vi "TrafficLight.vi"() -> ()   [LabVIEW 2018]
panel:
  in  "Car Waiting NS":bool
  in  "Car Waiting EW":bool
  in  "Light Time":sgl(slide)=1.0 min=1 max=30 step=1 scale=1.0..30.0
  in  "Flashing Red":bool
  in  "Emergency":bool
  out "NS2 G":bool
  out "NS2 Y":bool
  out "NS2 R":bool
  out "EW2 G":bool
  out "EW2 Y":bool
  out "EW2 R":bool
  out "NS1 G":bool
  out "NS1 Y":bool
  out "NS1 R":bool
  out "EW1 G":bool
  out "EW1 Y":bool
  out "EW1 R":bool
  in  "stop":bool
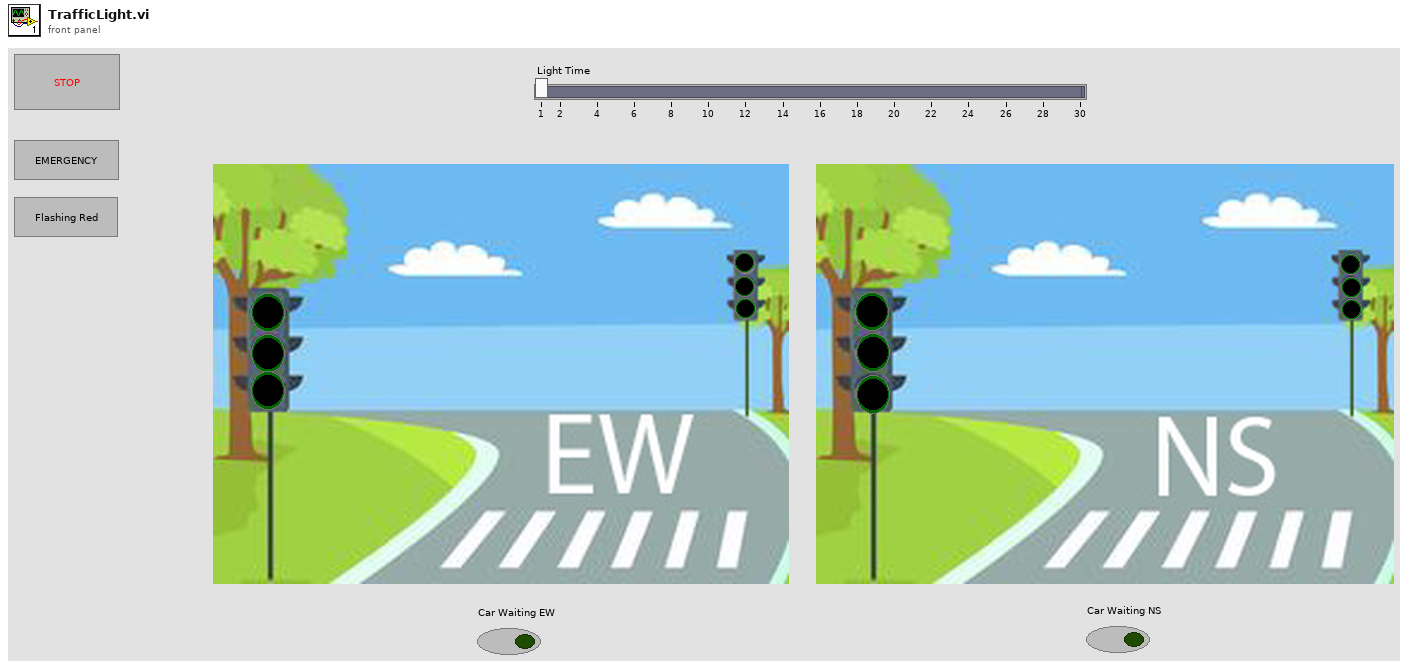
[diagram p1: front panel]
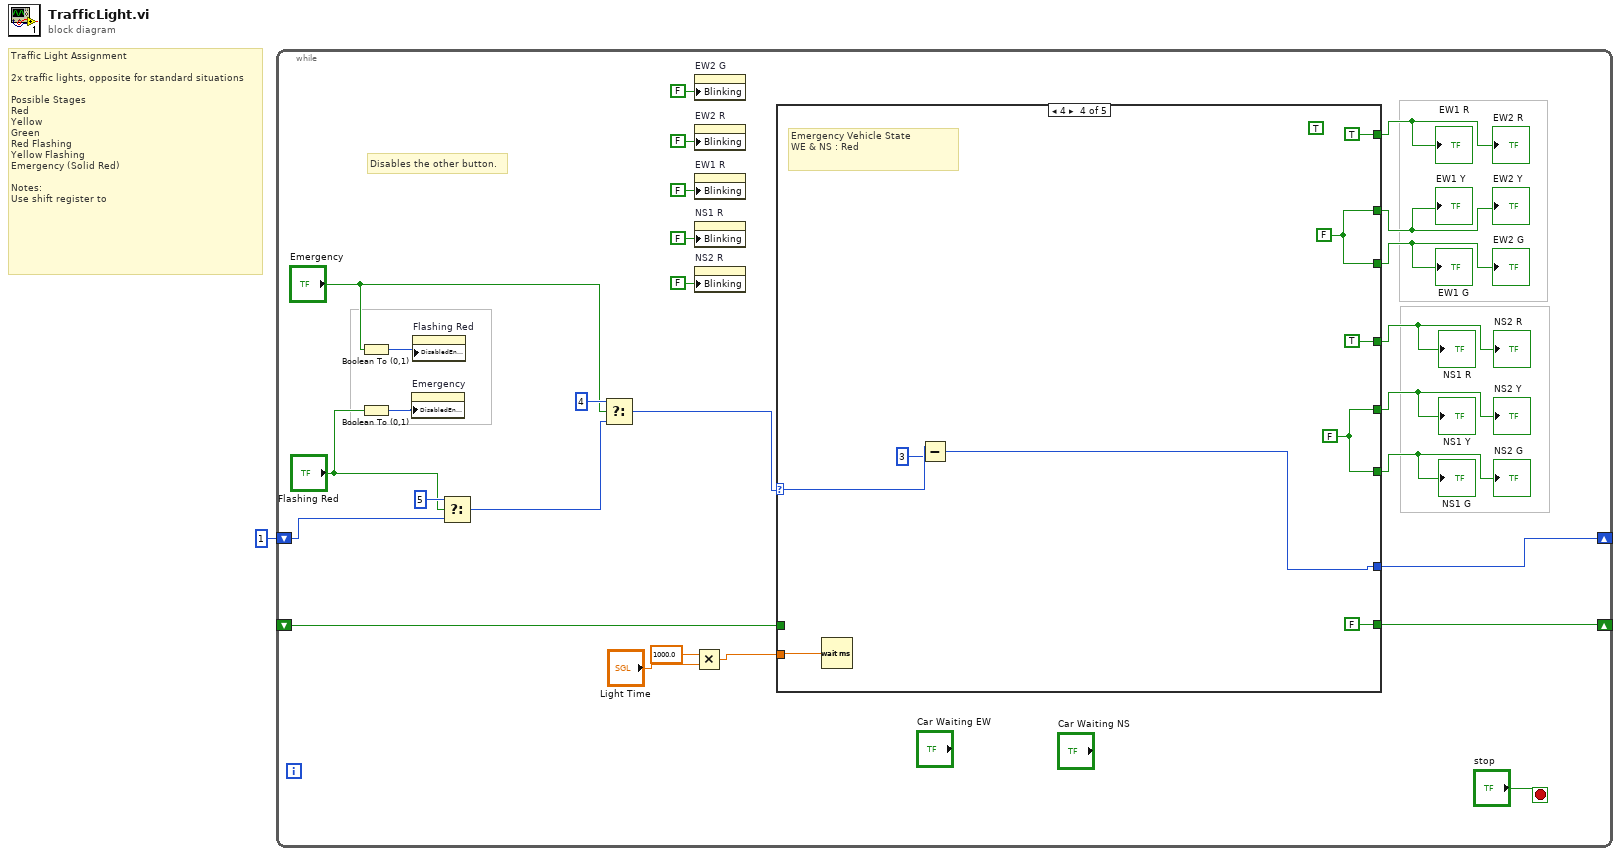
[diagram p0: block diagram]
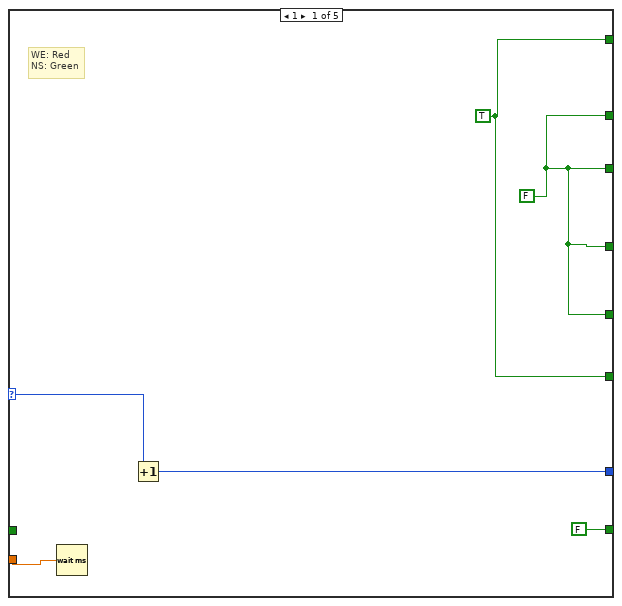
[diagram p2: hidden frame]
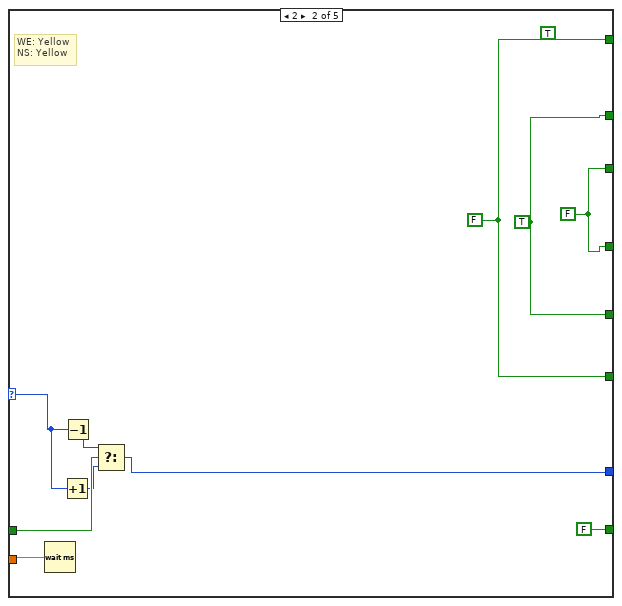
[diagram p3: hidden frame]
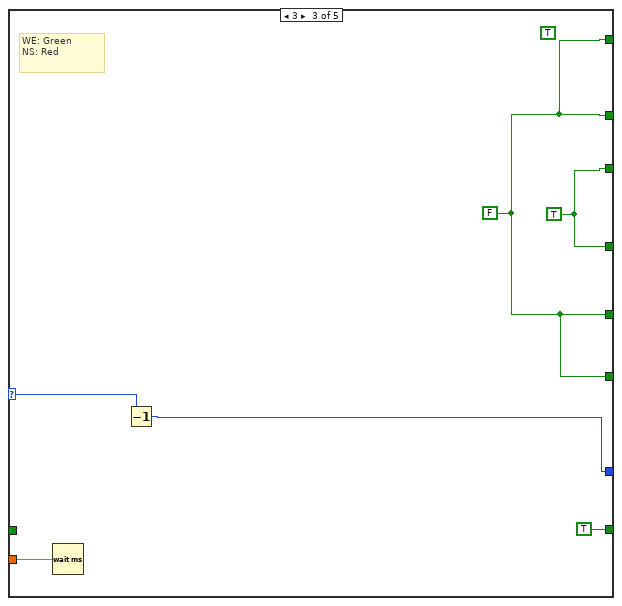
[diagram p4: hidden frame]
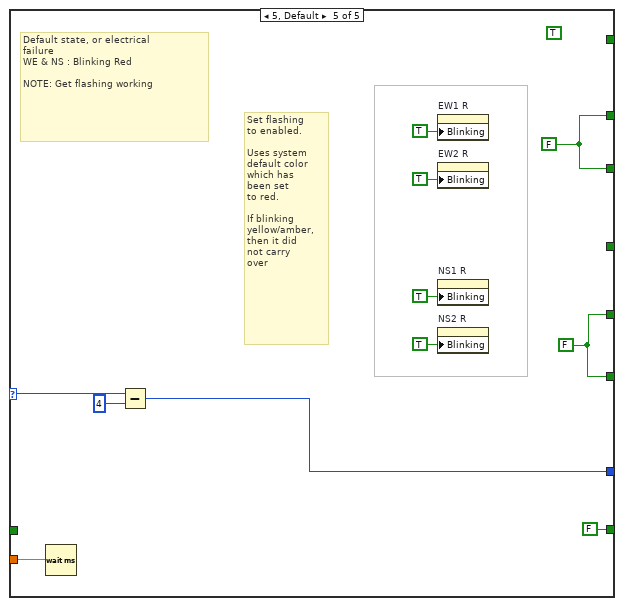
[diagram p5: hidden frame]
diagram:
  # "Traffic Light Assignment\n\n2x traffic lights, opposite for standard situations\n\nPossible Stages\nRed\nYellow\nGreen\nRed Flashing\nYellow Flashing\nEmergency (Solid Red)\n\nNotes:\nUse shift register to"
  n1 = while {
    shift-right: [w27] -> _
    shift-left: 1 -> [w18]
    shift-right: [w26] -> _
    shift-left: _ -> [w25]
    stop <- "stop" stop-if-true
    # "Disables the other button."
    n2 = Boolean To (0,1)(Boolean="Emergency") -> (0, 1=w11:i16)
    n3 = Boolean To (0,1)(Boolean="Flashing Red") -> (0, 1=w13:i16)
    n4 = property on="Emergency" class="Bool (strict)"("DisabledEnum"=w13) -> ()  [unwired: 2 in, 2 out]
    n5 = property on="Flashing Red" class="Bool (strict)"("DisabledEnum"=w11) -> ()  [unwired: 2 in, 2 out]
    n6 = Select(t=5, s="Flashing Red", f=w18) -> (s? t:f=w16:i32)
    n7 = Select(t=4, s="Emergency", f=w16) -> (s? t:f=w12:i32)
    n8 = Multiply(x=sgl 1000.0, y="Light Time") -> (x*y=w3:sgl)
    n9 = property on="EW2 G" class="Bool (strict)"("Blinking"=FALSE) -> ()  [unwired: 2 in, 2 out]
    n10 = property on="EW2 R" class="Bool (strict)"("Blinking"=FALSE) -> ()  [unwired: 2 in, 2 out]
    n11 = property on="EW1 R" class="Bool (strict)"("Blinking"=FALSE) -> ()  [unwired: 2 in, 2 out]
    n12 = property on="NS1 R" class="Bool (strict)"("Blinking"=FALSE) -> ()  [unwired: 2 in, 2 out]
    n13 = property on="NS2 R" class="Bool (strict)"("Blinking"=FALSE) -> ()  [unwired: 2 in, 2 out]
    n14 = case shown="4" w12 {
      selector: w12 -> [w32 w36 w48 w55 w68]
      tunnel: [w34 w43 w50 w57 w70] -> w22
      tunnel: [w34 w44 w49 w57 w70] -> w23
      tunnel: [w33 w42 w49 TRUE _] -> w24
      tunnel: [w34 w43 w50 TRUE _] -> w21
      tunnel: [w34 w44 w49 w56 w69] -> w20
      tunnel: [w33 w42 w49 w56 w69] -> w19
      tunnel: [w31 w39 w47 w53 w66] -> w27
      tunnel: [FALSE FALSE TRUE FALSE FALSE] -> w26
      tunnel: w25 -> [_ w40 _ _ _]
      tunnel: w3 -> [w29 w35 w45 w51 w60]
      frame 1 {
        w33 = TRUE
        w34 = FALSE
        # "WE: Red\nNS: Green"
        n15 = Wait (ms)(milliseconds to wait=w29) -> ()  [unwired: 1 out]
        n16 = Increment(x=w32) -> (x+1=w31:i32)
      }
      frame 2 {
        (unwired) TRUE ("Boolean")
        w42 = FALSE
        w43 = FALSE
        w44 = TRUE
        # "WE: Yellow\nNS: Yellow"
        n17 = Wait (ms)(milliseconds to wait=w35) -> ()  [unwired: 1 out]
        n18 = Increment(x=w36) -> (x+1=w37:i32)
        n19 = Decrement(x=w36) -> (x-1=w38:i32)
        n20 = Select(t=w38, s=w40, f=w37) -> (s? t:f=w39:i32)
      }
      frame 3 {
        (unwired) TRUE ("Boolean")
        w49 = FALSE
        w50 = TRUE
        # "WE: Green\nNS: Red"
        n21 = Wait (ms)(milliseconds to wait=w45) -> ()  [unwired: 1 out]
        n22 = Decrement(x=w48) -> (x-1=w47:i32)
      }
      frame 4 {
        (unwired) TRUE ("Boolean")
        w56 = FALSE
        w57 = FALSE
        # "Emergency Vehicle State\nWE & NS : Red"
        n23 = Wait (ms)(milliseconds to wait=w51) -> ()  [unwired: 1 out]
        n24 = Subtract(x=w55, y=3) -> (x-y=w53:i32)
      }
      frame 5, Default {
        (unwired) TRUE ("Boolean")
        w69 = FALSE
        w70 = FALSE
        # "Set flashing\nto enabled.\n\nUses system\ndefault color\nwhich has\nbeen set\nto red.\n\nIf blinking \nyellow/amber,\nthen it did\nnot carry \nover"
        # "Default state, or electrical\nfailure\nWE & NS : Blinking Red\n\nNOTE: Get flashing working"
        n25 = Wait (ms)(milliseconds to wait=w60) -> ()  [unwired: 1 out]
        n26 = Subtract(x=w68, y=4) -> (x-y=w66:i32)
        n27 = property on="EW1 R" class="Bool (strict)"("Blinking"=TRUE) -> ()  [unwired: 2 in, 2 out]
        n28 = property on="EW2 R" class="Bool (strict)"("Blinking"=TRUE) -> ()  [unwired: 2 in, 2 out]
        n29 = property on="NS1 R" class="Bool (strict)"("Blinking"=TRUE) -> ()  [unwired: 2 in, 2 out]
        n30 = property on="NS2 R" class="Bool (strict)"("Blinking"=TRUE) -> ()  [unwired: 2 in, 2 out]
      }
    }
    "EW1 R" <- w24
    "NS2 Y" <- w20
    "NS2 G" <- w19
    "EW2 G" <- w22
    "EW2 R" <- w24
    "EW2 Y" <- w23
    "NS1 Y" <- w20
    "NS1 G" <- w19
    "NS2 R" <- w21
    "EW1 G" <- w22
    "EW1 Y" <- w23
    "NS1 R" <- w21
  }
